vi "Parse Time.vi"(8 "error in (no error)":errorcluster, 11 "data":string) -> (0 "error out":errorcluster, 3 "Time Stamp":timestamp)   [LabVIEW 2018]
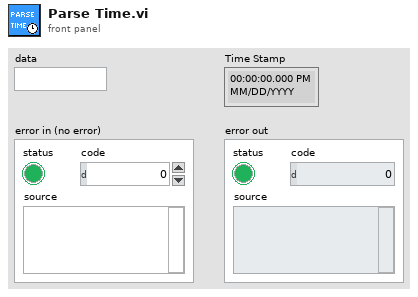
[diagram p1: front panel]
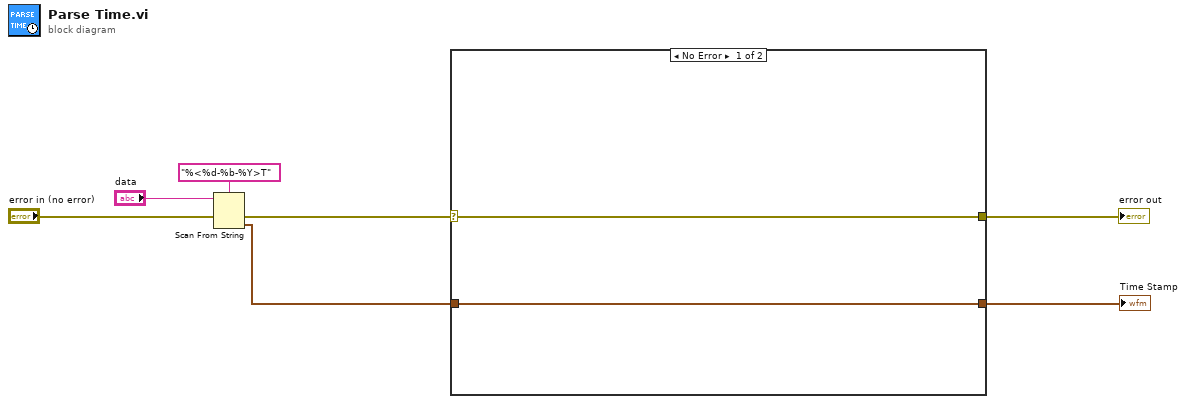
[diagram p0: block diagram]
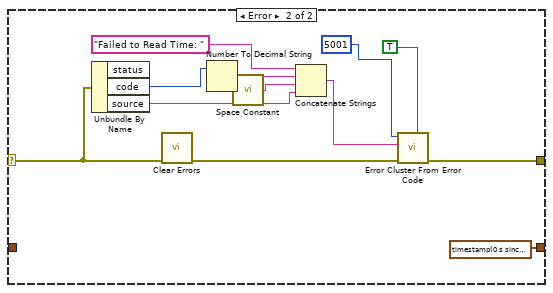
[diagram p2: hidden frame]
diagram:
  n1 = Scan From String(format string="%<%d-%b-%Y>T", input string="data", error in="error in (no error)") -> (error out=w4:errorcluster, output 1=w1:timestamp)  [unwired: 2 in, 2 out]
  n2 = case shown="No Error" w4 {
    selector: w4 -> [w9 w17]
    tunnel: [w9 w19] -> w3
    tunnel: [w8 timestamp(0 s since 1904-01-01)] -> w2
    tunnel: w1 -> [w8 _]
    frame No Error {
    }
    frame Error {
      n3 = Unbundle By Name(w17) -> ("code"=w14:i32, "source"=w13:string)  [unwired: 1 out]
      n4 = call <vilib>:"Clear Errors.vi"("error in (no error)"=w17) -> ("error out"=w18:errorcluster)  [unwired: 5 in, 1 out]
      n5 = Number To Decimal String(number=w14) -> (decimal integer string=w11:string)  [unwired: 1 in]
      n6 = call <vilib>:"Space Constant.vi"() -> ("String"=w12:string)
      n7 = Concatenate Strings("Failed to Read Time: " ("error message (\"\")"), w11, w12, w13) -> (w10:string)
      n8 = call <vilib>:"Error Cluster From Error Code.vi"("is warning? (False)"=TRUE, "error in (no error)"=w18, "error message (\"\")"=w10, "error code (0)"=5001) -> ("error out"=w19:errorcluster)  [unwired: 5 in]
    }
  }
  "error out" <- w3
  "Time Stamp" <- w2
